vi "Acquisition Message Loop.vi"(8 "error in (no error)":errorcluster, 9 "Data Queue":refnum<queue>, 10 "Data Notifier":refnum<notifier>, 11 "Message Queues":T1) -> (0 "error out":errorcluster)   [LabVIEW 2017, in "Acquisition.lvlib"]
doc: "Message loop for handling messages pertaining to the acquisition of data from the hardware."
uses:
  Acquisition.lvlib
  support/Message Queue/All Message Queues.ctl
  support/Message Queue/Message Cluster.ctl
  Hardware Configuration.ctl
  Signal Type.ctl
  Acquisition State.ctl
  support/Message Queue/Enqueue Message (Single).vi
  <vilib>/Utility/error.llb/Error Cluster From Error Code.vi
  <vilib>/ErrorRing/Error Ring.xnode
  support/Message Queue/Message Queue.lvlib
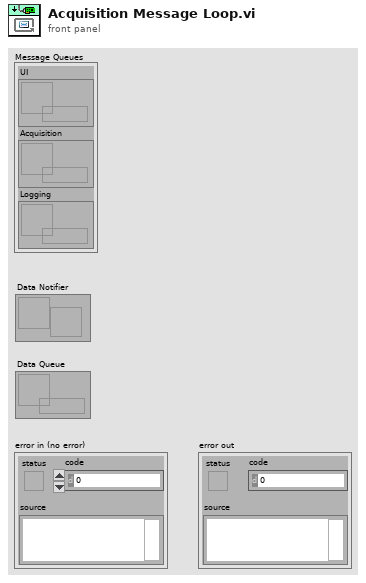
[diagram p1: front panel]
types:
  T1 = typedef "Message Queue.lvlib/All Message Queues.ctl" = cluster{"UI":refnum<queue>, "Acquisition":refnum<queue>, "Logging":refnum<queue>}
  T2 = typedef "Acquisition.lvlib/Hardware Configuration.ctl" = cluster{"HW Refnum <Replace Me>":string, "Signal Type <Replace Me>":T3}
  T3 = typedef "Acquisition.lvlib/Signal Type.ctl" = enum16{"Sine Wave", "Square with Noise"}
  T4 = typedef "Acquisition.lvlib/Acquisition State.ctl" = enum16{"Idle", "Acquiring"}
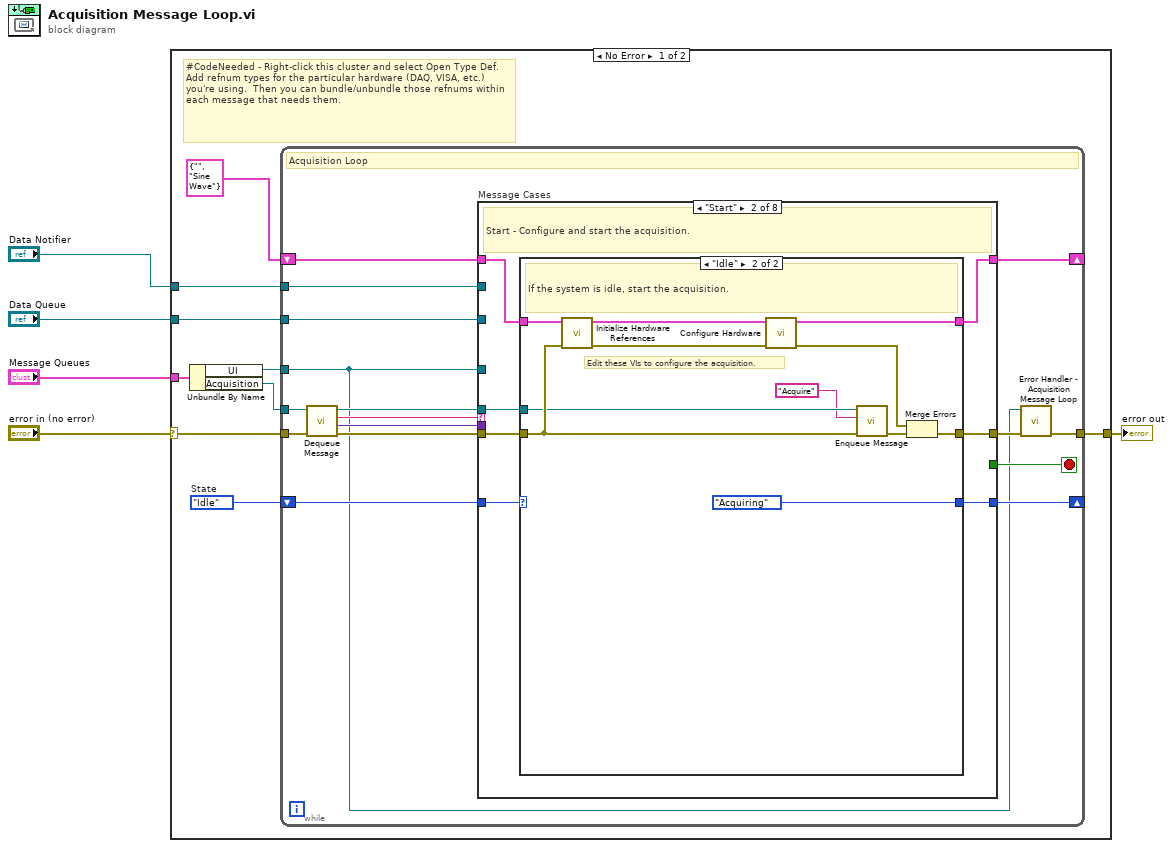
[diagram p0: block diagram]
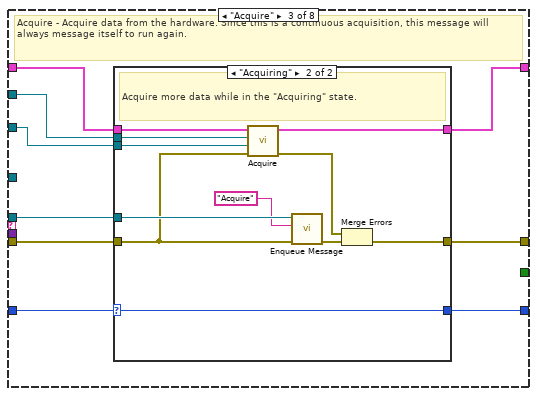
[diagram p4: hidden frame]
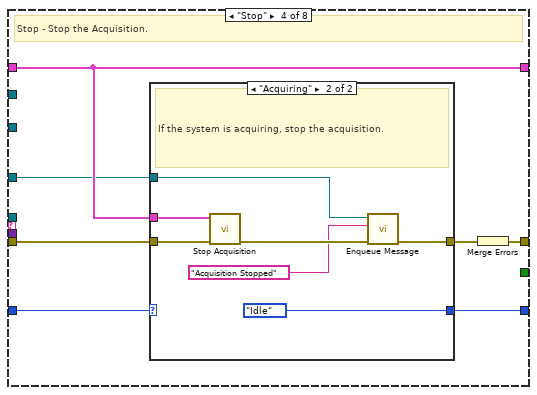
[diagram p6: hidden frame]
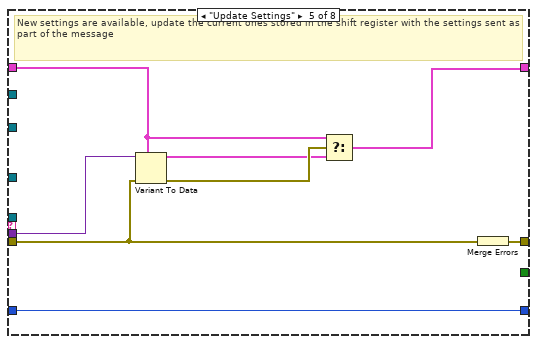
[diagram p8: hidden frame]
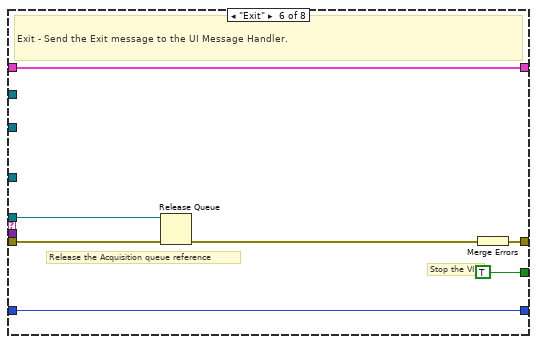
[diagram p9: hidden frame]
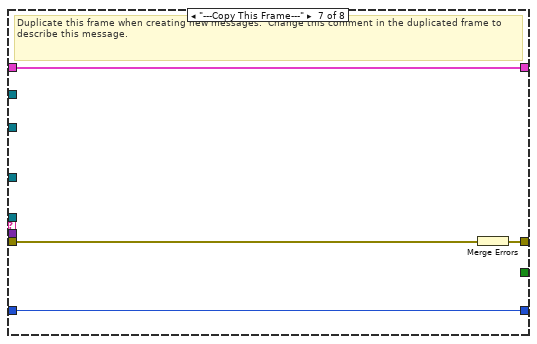
[diagram p10: hidden frame]
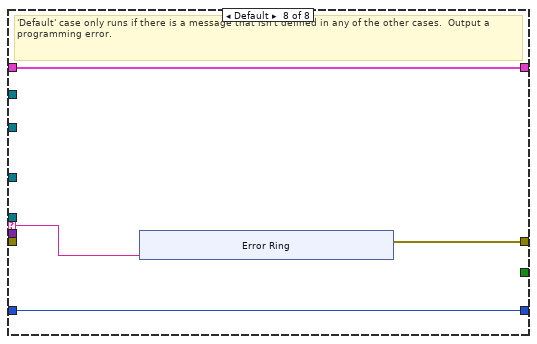
[diagram p11: hidden frame]
diagram:
  n1 = case shown="No Error" "error in (no error)" {
    selector: "error in (no error)" -> [w10 w124]
    tunnel: "Message Queues" -> [w14 _]
    tunnel: [w12 w124] -> w4
    tunnel: "Data Notifier" -> [w8 _]
    tunnel: "Data Queue" -> [w7 _]
    frame No Error {
      w6 = Acquisition_State."Idle"  # State
      # "#CodeNeeded - Right-click this cluster and select Open Type Def.  Add refnum types for the particular hardware (DAQ, VISA, etc.) you're using.  Then you can bundle/unbundle those refnums within each message that needs them."
      n2 = Unbundle By Name(w14) -> ("UI"=w9:refnum<queue>, "Acquisition"=w13:refnum<queue>)
      n3 = while {
        tunnel: w13 -> [w23]
        shift-right: [w29] -> _
        shift-left: T2 {"HW Refnum <Replace Me>"="", "Signal Type <Replace Me>"=enum."Sine Wave"} ("Data Cluster") -> [w30]
        tunnel: w9 -> [w15]
        tunnel: w8 -> [w22]
        tunnel: w7 -> [w21]
        shift-right: [w19] -> _
        shift-left: w6 -> [w20]
        tunnel: w10 -> [w27]
        tunnel: [w18] -> w12
        stop <- w28 stop-if-true
        # "Acquisition Loop"
        n4 = call "Dequeue Message.vi"("error in (no error)"=w27, "Message Queue"=w23) -> ("error out"=w26:errorcluster, "Message Data"=w24:variant, "Message"=w25:string, "dup Message Queue"=w16:refnum<queue>)  [unwired: 6 in]
        n5 = case "Message Cases" shown="\"Start\"" w25 {
          selector: w25 -> [_ _ _ _ _ _ _ w113]
          tunnel: w16 -> [_ w37 w62 _ _ w103 _ _]
          tunnel: w26 -> [w33 w38 w61 w83 w95 w105 w112 _]
          tunnel: [w33 w40 w63 w84 w101 w107 w110 w114] -> w17
          tunnel: w30 -> [w32 w39 w59 w81 w97 w106 w111 w116]
          tunnel: [w32 w36 w60 w81 w96 w106 w111 w116] -> w29
          tunnel: [_ _ _ _ _ TRUE _ _] -> w28
          tunnel: w24 -> [_ _ _ _ w100 _ _ _]
          tunnel: w15 -> [_ _ _ w78 _ _ _ _]
          tunnel: w22 -> [_ _ w58 _ _ _ _ _]
          tunnel: w21 -> [_ _ w57 _ _ _ _ _]
          tunnel: w20 -> [w31 w34 w55 w80 w94 w102 w109 w115]
          tunnel: [w31 w35 w56 w79 w94 w102 w109 w115] -> w19
          frame "Initialize" {
            # "Initialize  - Initialize is currently a no-op.  The hardware initialization takes place in the 'Start' message."
          }
          frame "Start" {
            # "Start - Configure and start the acquisition."
            n6 = case shown="\"Idle\"" w34 {
              selector: w34 -> [w41 _]
              tunnel: [w42 w54] -> w40
              tunnel: w39 -> [w43 w53]
              tunnel: w38 -> [w42 w52]
              tunnel: w37 -> [_ w50]
              tunnel: [w43 w46] -> w36
              tunnel: [w41 Acquisition_State."Acquiring" ("Acquisition State")] -> w35
              frame "Acquiring" {
                # "The system is already acquiring. Ignore the \"Start\" message."
              }
              frame "Idle" {
                # "Edit these VIs to configure the acquisition."
                # "If the system is idle, start the acquisition."
                n7 = call "Initialize Hardware References.vi"("error in (no error)"=w52, "Hardware Resources in"=w53) -> ("error out"=w49:errorcluster, "Hardware Resources out"=w47:T2)  [unwired: 8 in]
                n8 = call "Configure Hardware.vi"("error in (no error)"=w49, "Hardware Resources in"=w47) -> ("error out"=w48:errorcluster, "Hardware Resources out"=w46:T2)  [unwired: 8 in]
                n9 = call-poly "Enqueue Message.vi"("error in (no error)"=w52, "Message"="Acquire", "Message Queue"=w50) -> ("error out"=w51:errorcluster)  [unwired: 7 in, 1 out]
                n10 = Merge Errors(w48, w51) -> (w54:errorcluster)
              }
            }
          }
          frame "Acquire" {
            # "Acquire - Acquire data from the hardware. Since this is a continuous acquisition, this message will always message itself to run again."
            n11 = case shown="\"Acquiring\"" w55 {
              selector: w55 -> [w64 w68]
              tunnel: [w65 w77] -> w63
              tunnel: w62 -> [_ w75]
              tunnel: w61 -> [w65 w67]
              tunnel: [w66 w73] -> w60
              tunnel: w59 -> [w66 w72]
              tunnel: w58 -> [_ w70]
              tunnel: w57 -> [_ w69]
              tunnel: [w64 w68] -> w56
              frame "Idle" {
                # "Ignore \"Acquire\" messages when the acquisition is idle."
              }
              frame "Acquiring" {
                # "Acquire more data while in the \"Acquiring\" state."
                n12 = call "Acquire.vi"("error in (no error)"=w67, "Data Queue"=w69, "Data Notifier"=w70, "Hardware Resources in"=w72) -> ("error out"=w74:errorcluster, "Hardware Resources out"=w73:T2)  [unwired: 6 in]
                n13 = call-poly "Enqueue Message.vi"("error in (no error)"=w67, "Message"="Acquire", "Message Queue"=w75) -> ("error out"=w76:errorcluster)  [unwired: 7 in, 1 out]
                n14 = Merge Errors(w74, w76) -> (w77:errorcluster)
              }
            }
          }
          frame "Stop" {
            # "Stop - Stop the Acquisition."
            n15 = case shown="\"Acquiring\"" w80 {
              selector: w80 -> [w85 _]
              tunnel: w83 -> [w86 w93]
              tunnel: [w86 w89] -> w82
              tunnel: w81 -> [_ w91]
              tunnel: [w85 Acquisition_State."Idle" ("State")] -> w79
              tunnel: w78 -> [_ w88]
              frame "Idle" {
                # "The system is already idle. Ignore the \"Stop\" message."
              }
              frame "Acquiring" {
                # "If the system is acquiring, stop the acquisition."
                n16 = call "Stop Acquisition.vi"("error in (no error)"=w93, "Hardware Resources in"=w91) -> ("error out"=w92:errorcluster)  [unwired: 9 in]
                n17 = call-poly "Enqueue Message.vi"("error in (no error)"=w92, "Message"="Acquisition Stopped", "Message Queue"=w88) -> ("error out"=w89:errorcluster)  [unwired: 7 in, 1 out]
              }
            }
            n18 = Merge Errors(w82) -> (w84:errorcluster)
          }
          frame "Update Settings" {
            # "New settings are available, update the current ones stored in the shift register with the settings sent as part of the message"
            n19 = Variant To Data(error in=w95, type=w97, Variant=w100) -> (data=w98:T2, error out=w99:errorcluster)
            n20 = Select(t=w97, s=w99, f=w98) -> (s? t:f=w96:T2)
            n21 = Merge Errors(w95) -> (w101:errorcluster)
          }
          frame "Exit" {
            # "Release the Acquisition queue reference"
            # "Stop the VI"
            # "Exit - Send the Exit message to the UI Message Handler."
            n22 = Release Queue(queue=w103, error in (no error)=w105) -> (error out=w104:errorcluster)  [unwired: 1 in, 2 out]
            n23 = Merge Errors(w104) -> (w107:errorcluster)
          }
          frame "---Copy This Frame---" {
            # "Duplicate this frame when creating new messages.  Change this comment in the duplicated frame to describe this message."
            n24 = Merge Errors(w112) -> (w110:errorcluster)
          }
          frame Default {
            # "'Default' case only runs if there is a message that isn't defined in any of the other cases.  Output a programming error."
            n25 = xnode "Error Ring"("parameter 0"=w113) -> ("error out"=w114:errorcluster)
          }
        }
        n26 = call "Error Handler - Acquisition Message Loop.vi"("error in (no error)"=w17, "Message Queue"=w15) -> ("dup error in"=w18:errorcluster)  [unwired: 8 in, 1 out]
      }
    }
    frame Error {
    }
  }
  "error out" <- w4
